vi "playlist.vi"() -> ()   [LabVIEW 2012]
uses:
  System.Windows.Forms
  <vilib>/Utility/miscctls.llb/LVPoint32TypeDef.ctl
  <vilib>/Utility/error.llb/DialogType.ctl
  musicplayer_glo.vi
  <vilib>/Utility/inputDevices.llb/mouseAcquire.vi
  shell32.dll
  user32.dll
panel:
  out "file count":u32
  out "drop-array":string[](array[string])
  out "win msg queue":T1
  in  "cancel":bool
  in  "ProgressBar":refnum<k24>(container)
  out "verdeckung":bool=TRUE
  in  "playlist":i32[](listbox)=[-2] caption="Playlist"
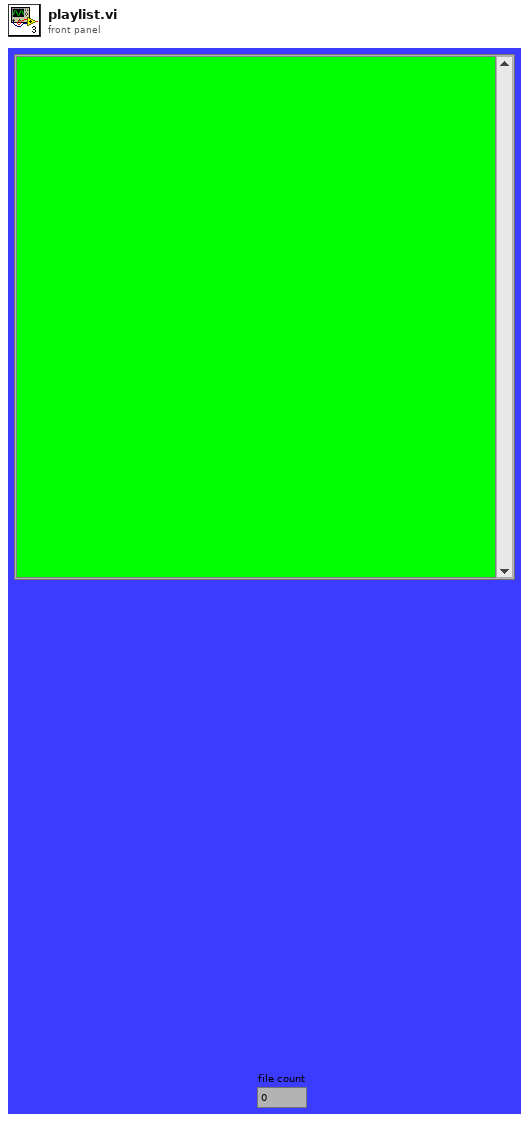
[diagram p1: front panel]
types:
  T1 = typedef "Win Msg Queue RefNum" = refnum<k1>
  T2 = enum8{"Enabled", "Disabled", "Disabled and Grayed Out"}
  T3 = enum32{"Invalid", "Standard", "Closed", "Hidden", "Minimized", "Maximized"}
  T4 = typedef "LVPoint32TypeDef.ctl" = cluster{"Horizontal":i32, "Vertical":i32}
  T5 = cluster{"Horizontal":i32, "Vertical":i32, "Scrolling":i32}
  T6 = cluster{"hWnd":u32, "Msg":u32, "wParam":u32, "lParam":i32, "time":u32, "point":cluster{"X":i32, "Y":i32}}
  T7 = typedef "DialogType.ctl" = u16
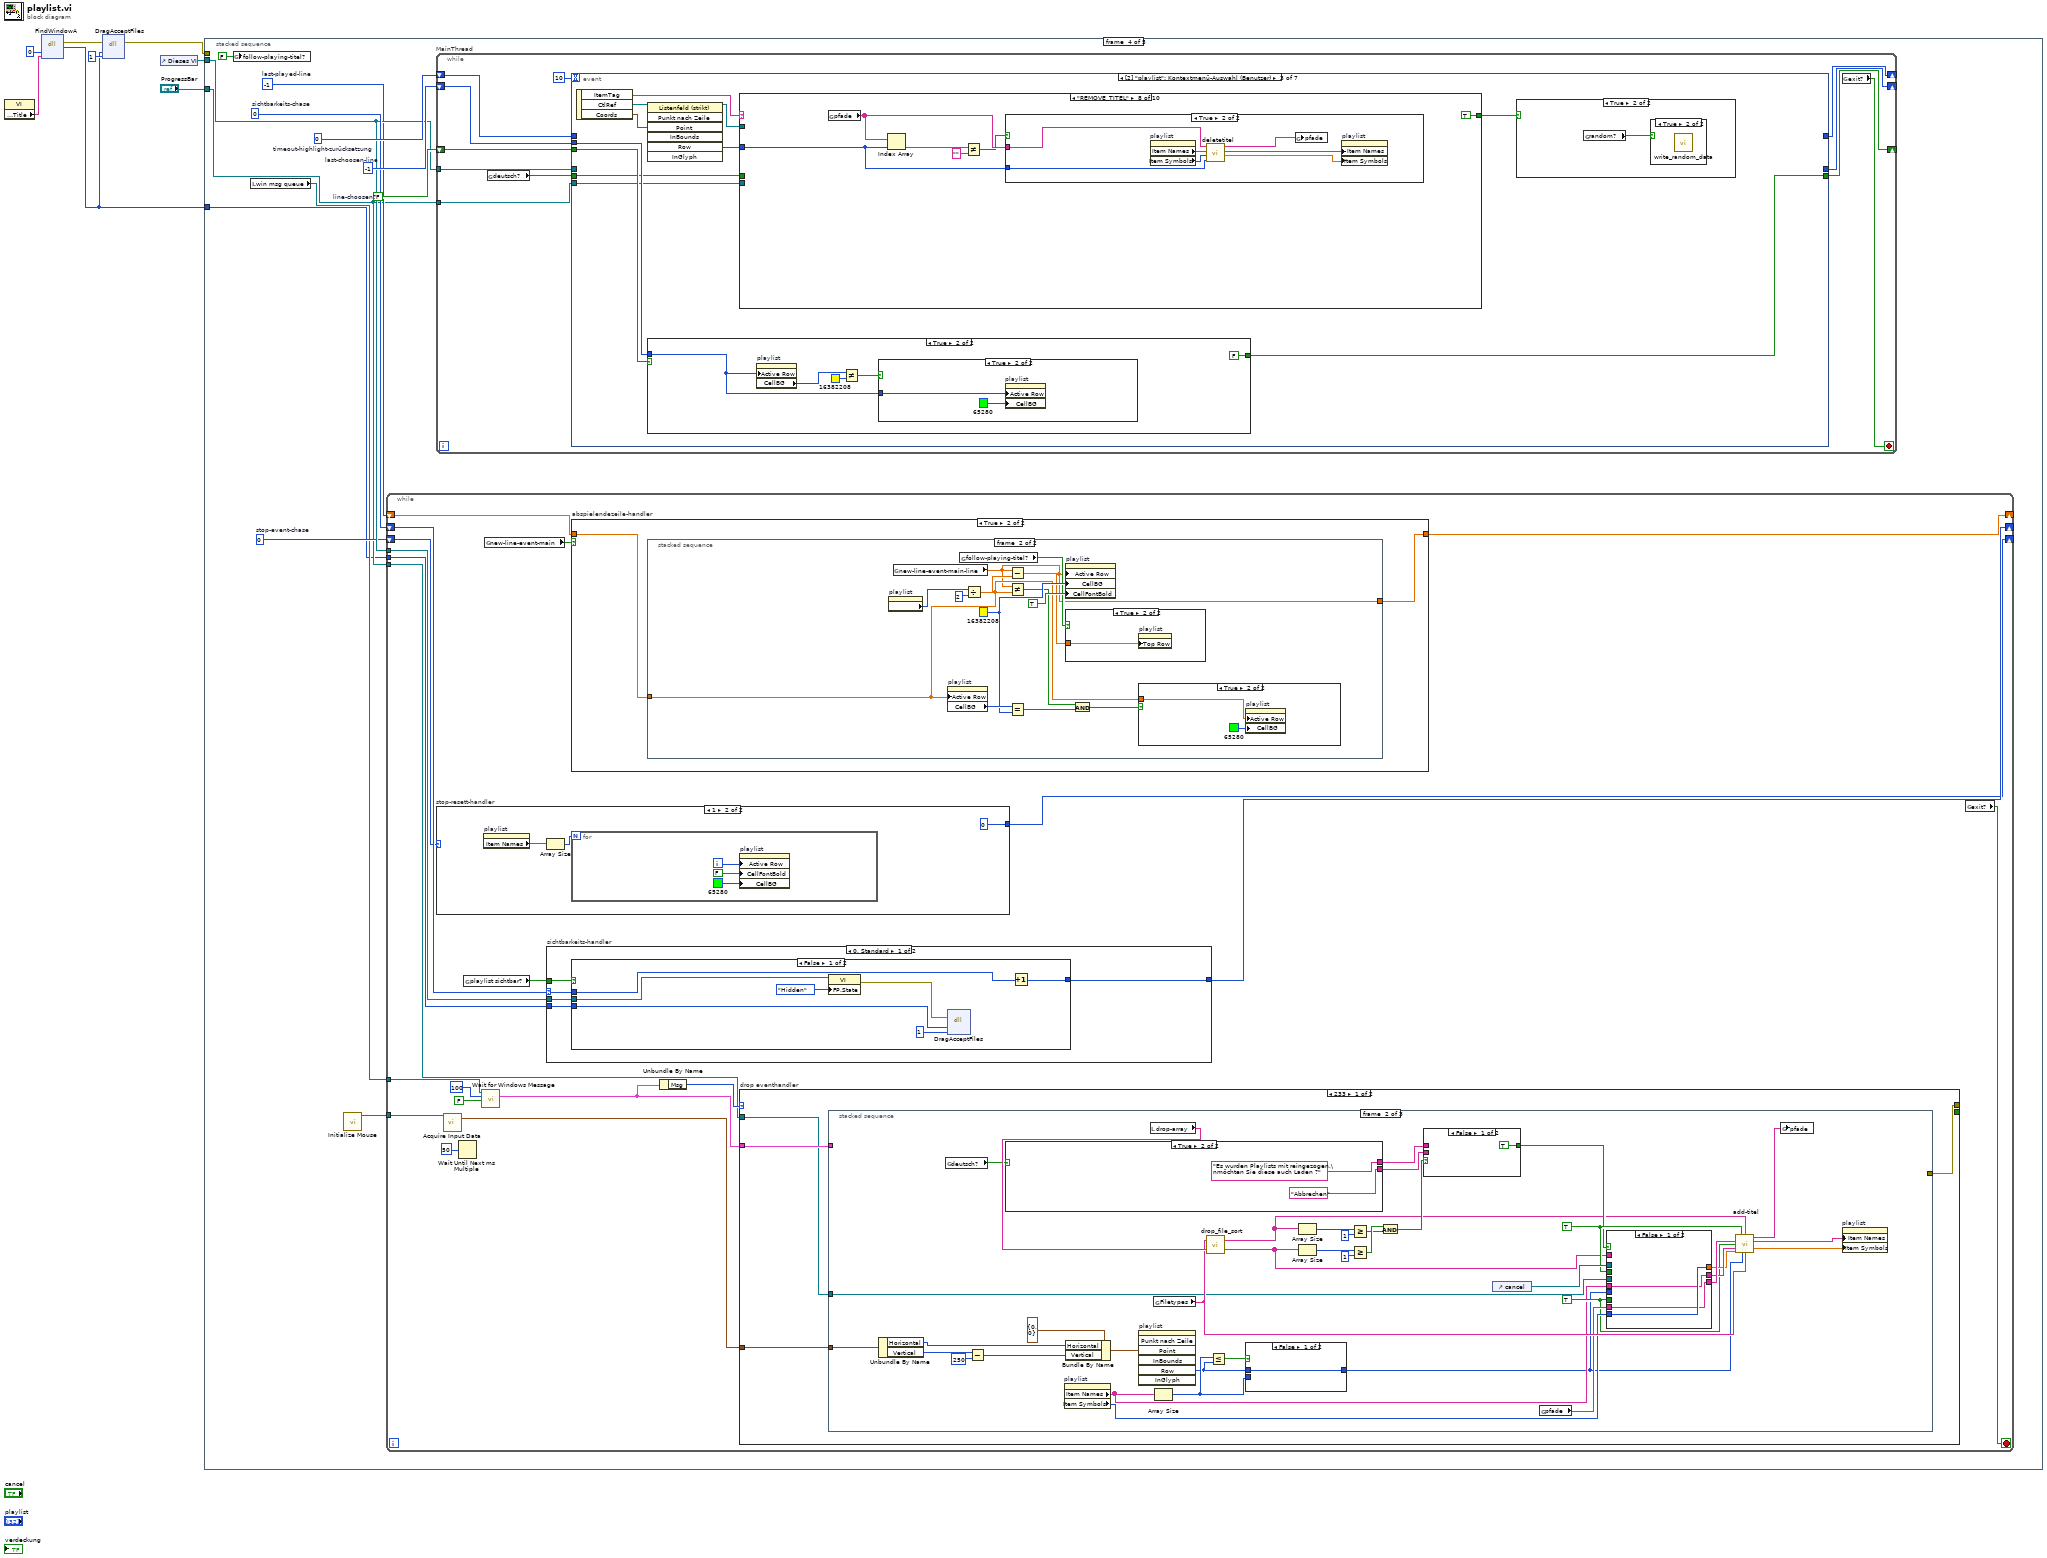
[diagram p0: block diagram]
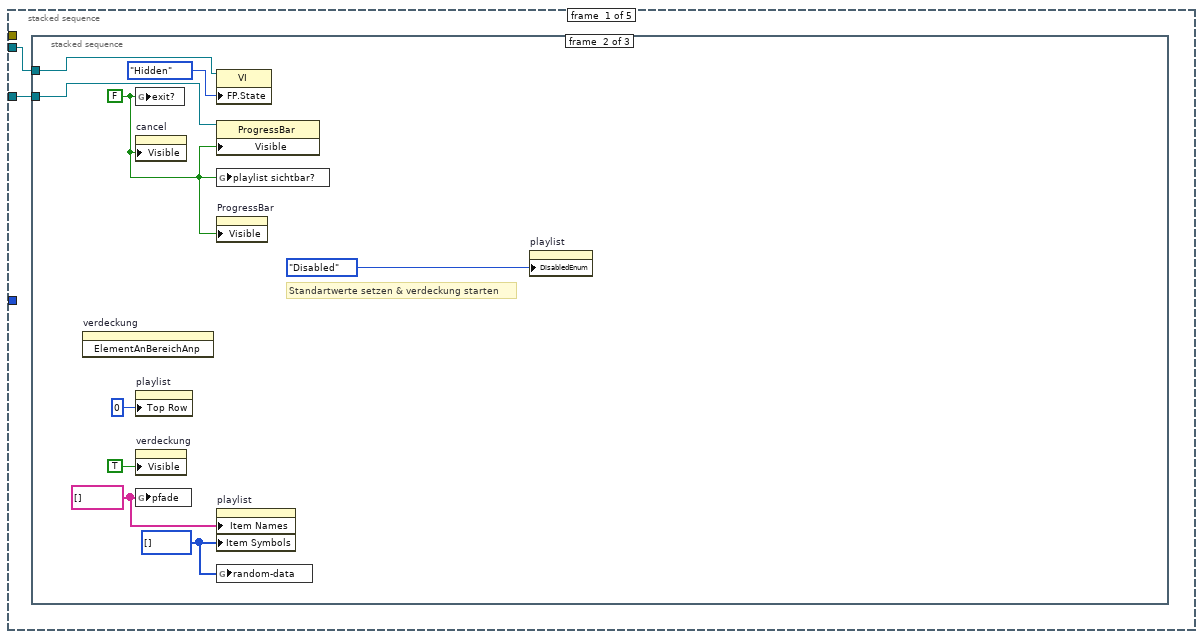
[diagram p2: hidden frame]
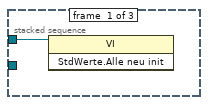
[diagram p3: hidden frame]
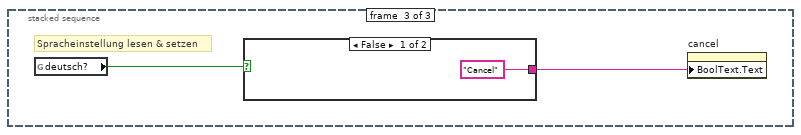
[diagram p4: hidden frame]
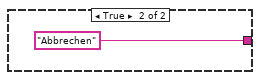
[diagram p5: hidden frame]
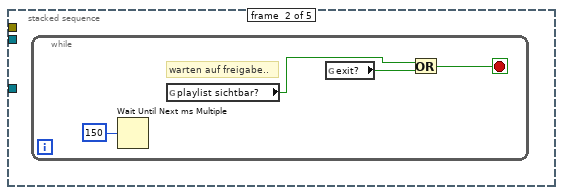
[diagram p6: hidden frame]
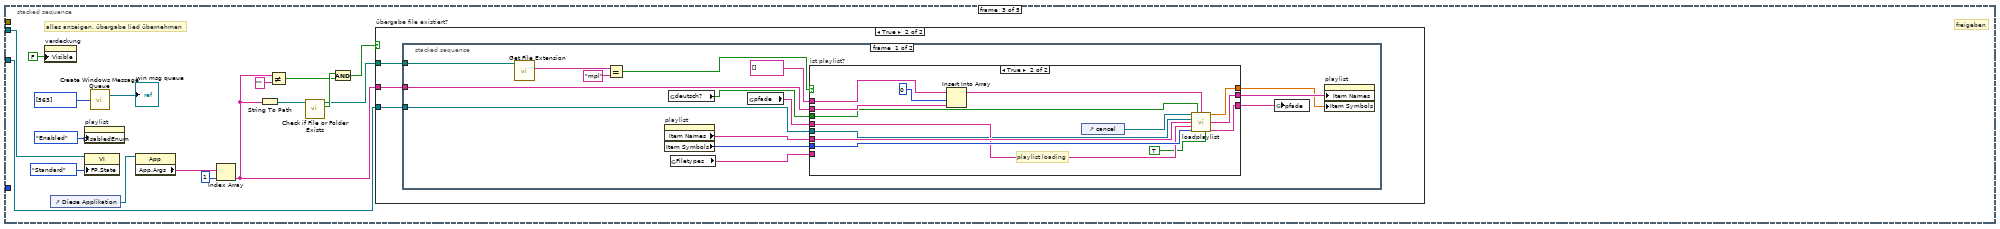
[diagram p7: hidden frame]
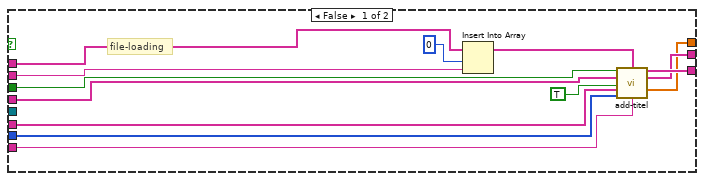
[diagram p9: hidden frame]
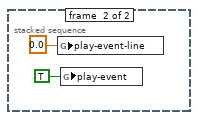
[diagram p10: hidden frame]
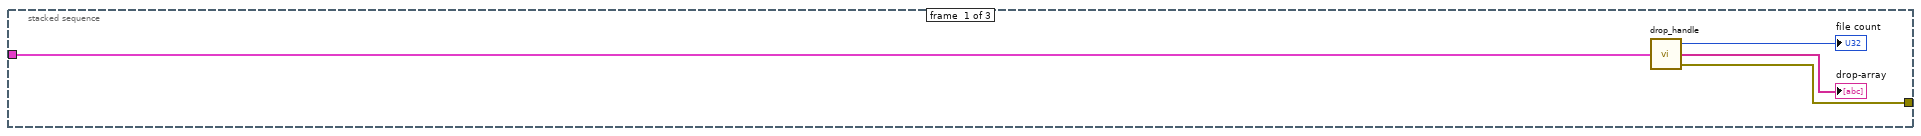
[diagram p11: hidden frame]
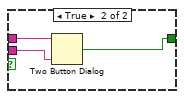
[diagram p12: hidden frame]
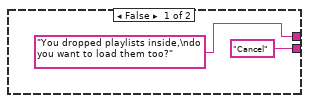
[diagram p13: hidden frame]
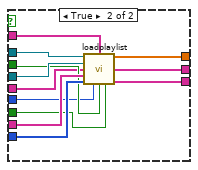
[diagram p14: hidden frame]
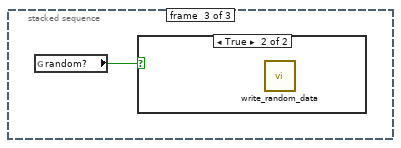
[diagram p16: hidden frame]
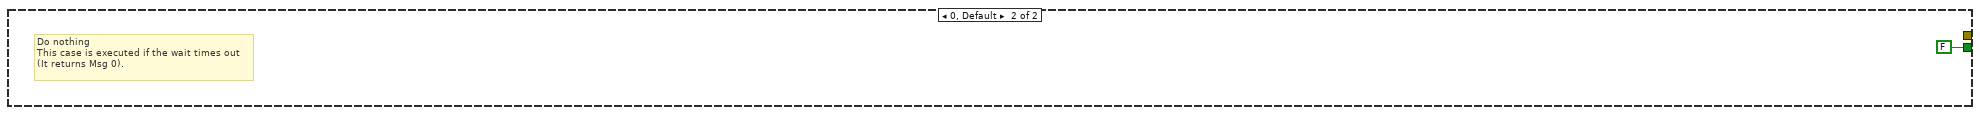
[diagram p18: hidden frame]
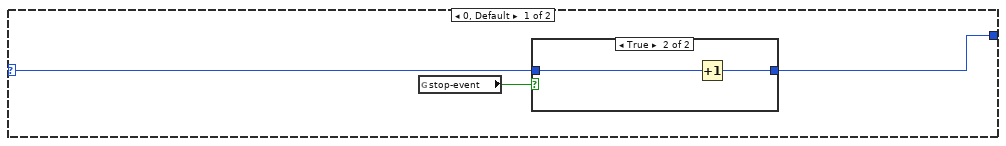
[diagram p19: hidden frame]
diagram:
  n1 = property class="VI"() -> ("Front Panel Window:Title"=w5:string)  [unwired: 2 in, 2 out]
  n2 = dll-call lib="user32.dll" fn="FindWindowA" label="FindWindow"("lpszClassName"=0, "lpszWindowName"=w5) -> (error out=w6:errorcluster, "hWnd"=w1:u32)  [unwired: 5 in, 1 out]
  n3 = dll-call lib="shell32.dll" fn="DragAcceptFiles"(error in=w6, "hWnd"=w1, "fAccept"=1) -> (error out=w2:errorcluster)  [unwired: 5 in, 1 out]
  n4 = control-ref of="Dieses VI"() -> (w8:refnum<vi>)
  n5 = stacked-sequence {
    tunnel: w8 -> [w10 _ w43 w99 w433]
    tunnel: "ProgressBar" -> [w9 _ w29 w94 _]
    tunnel: w2 -> [_ _ _ _ _]
    tunnel: w1 -> [_ _ _ w93 _]
    frame #0 {
      n6 = stacked-sequence {
        tunnel: w10 -> [w11 w17 _]
        tunnel: w9 -> [_ w15 _]
        frame #0 {
          n7 = invoke class="VI" method="StdWerte.Alle neu init"(reference=w11) -> ()  [unwired: 2 in, 3 out]
        }
        frame #1 {
          w12 = i32[] []
          w13 = string[] []
          w14 = FALSE ("playlist sichtbar?")
          # "Standartwerte setzen & verdeckung starten"
          n8 = invoke on="verdeckung" class="Bool." method="ElementAnBereichAnp"() -> ()  [unwired: 3 in, 3 out]
          n9 = global write "musicplayer_glo.vi" "exit?"(w14) -> ()
          n10 = property on="cancel" class="Bool. (strikt)"("Visible"=w14) -> ()  [unwired: 2 in, 2 out]
          n11 = property on="playlist" class="Listenfeld (strikt)"("Top Row"=0 ("Erste Zeile")) -> ()  [unwired: 2 in, 2 out]
          n12 = property on="verdeckung" class="Bool."("Visible"=TRUE ("Sichtbar")) -> ()  [unwired: 2 in, 2 out]
          n13 = global write "musicplayer_glo.vi" "pfade"(w13) -> ()
          n14 = property class="VI"(reference=w17, "FP.State"=T3."Hidden" ("Frontpanel-Fenster:Status")) -> ()  [unwired: 1 in, 2 out]
          n15 = property class="ProgressBar"(reference=w15, "Visible"=w14) -> ()  [unwired: 1 in, 2 out]
          n16 = global write "musicplayer_glo.vi" "playlist sichtbar?"(w14) -> ()
          n17 = property on="ProgressBar" class="AXCont"("Visible"=w14) -> ()  [unwired: 2 in, 2 out]
          n18 = property on="playlist" class="Listenfeld (strikt)"("Item Names"=w13, "Item Symbols"=w12) -> ()  [unwired: 2 in, 2 out]
          n19 = global write "musicplayer_glo.vi" "random-data"(w12) -> ()
          n20 = property on="playlist" class="Listenfeld (strikt)"("DisabledEnum"=T2."Disabled" ("Deaktiviert")) -> ()  [unwired: 2 in, 2 out]
        }
        frame #2 {
          # "Spracheinstellung lesen & setzen"
          n21 = global read "musicplayer_glo.vi" "deutsch?"() -> (w22:bool)
          n22 = case shown="False" w22 {
            tunnel: ["Cancel" "Abbrechen"] -> w21
            frame False {
            }
            frame True {
            }
          }
          n23 = property on="cancel" class="Bool. (strikt)"("BoolText.Text"=w21) -> ()  [unwired: 2 in, 2 out]
        }
      }
    }
    frame #1 {
      n24 = while {
        stop <- w26 stop-if-true
        # "warten auf freigabe.."
        n25 = Wait Until Next ms Multiple(millisecond multiple=u32 150 ("Vielfache von ms")) -> ()  [unwired: 1 out]
        n26 = global read "musicplayer_glo.vi" "playlist sichtbar?"() -> (w27:bool)
        n27 = global read "musicplayer_glo.vi" "exit?"() -> (w25:bool)
        n28 = Or(x=w27, y=w25) -> (x .or. y?=w26:bool)
      }
    }
    frame #2 {
      # "alles anzeigen, übergabe lied übernehmen"
      # "freigeben"
      n29 = property on="verdeckung" class="Bool."("Visible"=FALSE ("Sichtbar")) -> ()  [unwired: 2 in, 2 out]
      n30 = control-ref of="Diese Applikation"() -> (w39:refnum<vi>)
      n31 = property on="playlist" class="Listenfeld (strikt)"("DisabledEnum"=T2."Enabled" ("Deaktiviert")) -> ()  [unwired: 2 in, 2 out]
      n32 = property class="VI"(reference=w43, "FP.State"=T3."Standard" ("Frontpanel-Fenster:Status")) -> ()  [unwired: 1 in, 2 out]
      n33 = call "Create Windows Message Queue.vi"("Messeges (none)"=u32[] [563]) -> ("win msg queue"=→"win msg queue":T1)  [unwired: 2 in, 1 out]
      n34 = property class="App"(reference=w39) -> ("App.Args"=w38:string[])  [unwired: 1 in, 2 out]
      n35 = Index Array(array=w38, index=1 ("Index")) -> (element=w33:string)
      n36 = String To Path(string=w33) -> (path=w36:path)
      n37 = Not Equal?(x=w33, y="") -> (x != y?=w30:bool)
      n38 = call <vilib>:"Check if File or Folder Exists.vi"("path"=w36) -> ("file or folder exists?"=w35:bool, "dup path"=w34:path)  [unwired: 8 in, 1 out]
      n39 = And(x=w35, y=w30) -> (x .and. y?=w31:bool)
      n40 = case "übergabe file existiert?" shown="True" w31 {
        tunnel: w34 -> [_ w48]
        tunnel: w33 -> [_ w47]
        tunnel: w29 -> [_ w46]
        frame False {
        }
        frame True {
          n41 = stacked-sequence {
            tunnel: w48 -> [w63 _]
            tunnel: w47 -> [w55 _]
            tunnel: w46 -> [w49 _]
            frame #0 {
              n42 = call <vilib>:"Get File Extension.vi"("file"=w63) -> ("lowercase file extension"=w62:string)  [unwired: 7 in, 3 out]
              n43 = Equal?(x=w62, y="mpl") -> (x = y?=w60:bool)
              n44 = property on="playlist" class="Listenfeld (strikt)"() -> ("Item Names"=w57:string[], "Item Symbols"=w56:i32[])  [unwired: 2 in, 2 out]
              n45 = global read "musicplayer_glo.vi" "deutsch?"() -> (w59:bool)
              n46 = global read "musicplayer_glo.vi" "Filetypes"() -> (w54:string)
              n47 = global read "musicplayer_glo.vi" "pfade"() -> (w58:string[])
              n48 = case "ist playlist?" shown="True" w60 {
                tunnel: w59 -> [w76 w86]
                tunnel: w58 -> [w75 w83]
                tunnel: w57 -> [w73 w85]
                tunnel: w56 -> [w72 w84]
                tunnel: w55 -> [w70 w88]
                tunnel: w54 -> [w68 _]
                tunnel: [w67 w81] -> w53
                tunnel: [w66 w80] -> w52
                tunnel: [w65 w79] -> w51
                tunnel: string[] [] -> [w64 w89]
                tunnel: w49 -> [_ w78]
                frame False {
                  # "file-loading"
                  n49 = Insert Into Array(array=w64, index=0 ("Index"), new element=w70) -> (w69:string[])
                  n50 = call "add-titel.vi"("deutsch?"=w76, "input-array"=w69, "pfade"=w75, "use input-array?"=TRUE, "playlist"=w73, "symbole"=w72, "dateitypen"=w68) -> ("pfade out"=w67:string[], "playlist out"=w66:string[], "symbole out"=w65:dbl[])  [unwired: 6 in]
                }
                frame True {
                  # "playlist loading"
                  n51 = Insert Into Array(array=w89, index=0 ("Index"), new element=w88) -> (w87:string[])
                  n52 = control-ref of="cancel"() -> (w77:refnum<vi>)
                  n53 = call "loadplaylist.vi"("Boolesch-ref"=w77, "deutsch?"=w86, "input-array"=w87, "ProgressBar-ref"=w78, "playlist-input"=w85, "pfade-in"=w83, "symbole-in"=w84, "von input-array?"=TRUE) -> ("symbole-out"=w79:dbl[], "playlist-output"=w80:string[], "pfade-out"=w81:string[])  [unwired: 5 in]
                }
              }
              n54 = global write "musicplayer_glo.vi" "pfade"(w53) -> ()
              n55 = property on="playlist" class="Listenfeld (strikt)"("Item Names"=w52, "Item Symbols"=w51) -> ()  [unwired: 2 in, 2 out]
            }
            frame #1 {
              n56 = global write "musicplayer_glo.vi" "play-event-line"(0.0 ("play-event-line")) -> ()
              n57 = global write "musicplayer_glo.vi" "play-event"(TRUE ("play-event-playlist")) -> ()
            }
          }
        }
      }
    }
    frame #3 {
      w97 = 0  # stop-event-chase
      w98 = -1  # last-played-line
      w100 = 0  # sichtbarkeits-chase
      w102 = 0  # timeout-highlight-zurücksetzung
      w103 = FALSE  # line-choosen?
      w104 = -1  # last-choosen-line
      n58 = global write "musicplayer_glo.vi" "follow-playing-titel?"(FALSE ("follow-playing-titel?")) -> ()
      n59 = local read "win msg queue"() -> (w96:T1)
      n60 = call <vilib>:"Initialize Mouse.vi"() -> ("device ID"=w95:refnum<k1>)  [unwired: 10 in, 1 out]
      n61 = while {
        shift-right: [w120] -> _
        shift-left: w100 -> [w122]
        tunnel: w99 -> [w121]
        shift-right: [w117] -> _
        shift-left: w98 -> [w118]
        shift-right: [w115] -> _
        shift-left: w97 -> [w116]
        tunnel: w96 -> [w109]
        tunnel: w95 -> [w108]
        tunnel: w94 -> [w107]
        tunnel: w93 -> [w105]
        stop <- w106 stop-if-true
        n62 = case "stop-resett-handler" shown="1" w116 {
          selector: w116 -> [w200 _]
          tunnel: [w199 0] -> w115
          frame 0, Default {
            n63 = global read "musicplayer_glo.vi" "stop-event"() -> (w201:bool)
            n64 = case shown="True" w201 {
              tunnel: w200 -> [w202 w204]
              tunnel: [w202 w203] -> w199
              frame False {
              }
              frame True {
                n65 = Increment(x=w204) -> (x+1=w203:i32)
              }
            }
          }
          frame 1 {
            n66 = property on="playlist" class="Listenfeld (strikt)"() -> ("Item Names"=w207:string[])  [unwired: 2 in, 2 out]
            n67 = Array Size(array=w207) -> (size(s)=w206:i32)
            n68 = for {
              N: w206 -> [_]
              i -> [w209]
              n69 = property on="playlist" class="Listenfeld (strikt)"("Active Row"=w209, "CellFontBold"=FALSE ("Aktive Zeile:Schriftart der Zelle:Fett"), "CellBG"=u32 65280 ("Farbfeld 2")) -> ()  [unwired: 2 in, 2 out]
            }
          }
        }
        n70 = call-poly <vilib>:"Acquire Input Data.vi"("device ID"=w108) -> ("axis info"=w112:T5)  [unwired: 15 in, 3 out]
        n71 = Wait Until Next ms Multiple(millisecond multiple=u32 50 ("Vielfache von ms")) -> ()  [unwired: 1 out]
        n72 = global read "musicplayer_glo.vi" "playlist sichtbar?"() -> (w123:bool)
        n73 = call "Wait for Windows Message.vi"("win msg queue"=w109, "ms timeout (-1)"=100, "ignore previous (F)"=FALSE ("ignore previous (T)")) -> ("Message"=w111:T6)  [unwired: 1 in, 5 out]
        n74 = global read "musicplayer_glo.vi" "new-line-event-main"() -> (w119:bool)
        n75 = case "sichtbarkeits-handler" shown="0, Standard" w122 {
          selector: w122 -> [w234 w246]
          tunnel: w123 -> [w235 w248]
          tunnel: [w233 w247] -> w120
          tunnel: w121 -> [w232 w245]
          tunnel: w105 -> [w231 w244]
          frame 0, Default {
            n76 = case shown="False" w235 {
              tunnel: w234 -> [w240 w243]
              tunnel: [w239 w243] -> w233
              tunnel: w232 -> [w242 _]
              tunnel: w231 -> [w237 _]
              frame False {
                n77 = property class="VI"(reference=w242, "FP.State"=T3."Hidden" ("Frontpanel-Fenster:Status")) -> (error out=w236:errorcluster)  [unwired: 1 in, 1 out]
                n78 = dll-call lib="shell32.dll" fn="DragAcceptFiles"(error in=w236, "hWnd"=w237, "fAccept"=1) -> ()  [unwired: 5 in, 2 out]
                n79 = Increment(x=w240) -> (x+1=w239:i32)
              }
              frame True {
              }
            }
          }
          frame 1 {
            n80 = case shown="True" w248 {
              tunnel: [w249 0] -> w247
              tunnel: w246 -> [w249 _]
              tunnel: w245 -> [_ w253]
              tunnel: w244 -> [_ w251]
              frame False {
              }
              frame True {
                n81 = property class="VI"(reference=w253, "FP.State"=T3."Standard" ("Frontpanel-Fenster:Status")) -> (error out=w250:errorcluster)  [unwired: 1 in, 1 out]
                n82 = dll-call lib="shell32.dll" fn="DragAcceptFiles"(error in=w250, "hWnd"=w251, "fAccept"=1) -> ()  [unwired: 5 in, 2 out]
              }
            }
          }
        }
        n83 = case "abspielendezeile-handler" shown="True" w119 {
          tunnel: w118 -> [w211 w213]
          tunnel: [w211 w212] -> w117
          frame False {
          }
          frame True {
            n84 = stacked-sequence {
              tunnel: w213 -> [_ w216]
              tunnel: [_ w215] -> w212
              frame #0 {
                n85 = global write "musicplayer_glo.vi" "new-line-event-main"(FALSE ("new-line-event-main")) -> ()
              }
              frame #1 {
                w223 = u32 16382208 ("Farbfeld 2")
                n86 = property on="playlist" class="Listenfeld (strikt)"() -> ("Number of Rows"=w221:u32)  [unwired: 2 in, 2 out]
                n87 = global read "musicplayer_glo.vi" "new-line-event-main-line"() -> (w215:dbl)
                n88 = property on="playlist" class="Listenfeld (strikt)"("Active Row"=w216) -> ("CellBG"=w227:u32)  [unwired: 2 in, 2 out]
                n89 = global read "musicplayer_glo.vi" "follow-playing-titel?"() -> (w218:bool)
                n90 = Divide(x=w221, y=u32 2) -> (x/y=w217:dbl)
                n91 = Subtract(x=w215, y=w217) -> (x-y=w219:dbl)
                n92 = Not Equal?(x=w215, y=w216) -> (x != y?=w222:bool)
                n93 = Equal?(x=w227, y=w223) -> (x = y?=w226:bool)
                n94 = property on="playlist" class="Listenfeld (strikt)"("Active Row"=w215, "CellBG"=w223, "CellFontBold"=TRUE ("Aktive Zeile:Schriftart der Zelle:Fett")) -> ()  [unwired: 2 in, 2 out]
                n95 = case shown="True" w218 {
                  tunnel: w219 -> [_ w228]
                  frame False {
                  }
                  frame True {
                    n96 = property on="playlist" class="Listenfeld (strikt)"("Top Row"=w228) -> ()  [unwired: 2 in, 2 out]
                  }
                }
                n97 = And(x=w222, y=w226) -> (x .and. y?=w224:bool)
                n98 = case shown="True" w224 {
                  tunnel: w216 -> [_ w230]
                  frame False {
                  }
                  frame True {
                    n99 = property on="playlist" class="Listenfeld (strikt)"("Active Row"=w230, "CellBG"=u32 65280 ("Farbfeld 2")) -> ()  [unwired: 2 in, 2 out]
                  }
                }
              }
            }
          }
        }
        n100 = Unbundle By Name(w111) -> ("Msg"=w110:u32)
        n101 = case "drop eventhandler" shown="233" w110 {
          tunnel: [_ FALSE] -> _
          tunnel: [w127 _] -> _
          tunnel: w111 -> [w128 _]
          tunnel: w107 -> [w126 _]
          tunnel: w112 -> [w125 _]
          frame 563 {
            n102 = stacked-sequence {
              tunnel: [w132 _ _] -> w127
              tunnel: w128 -> [w131 _ _]
              tunnel: w126 -> [_ w165 _]
              tunnel: w125 -> [_ w146 _]
              frame #0 {
                n103 = call "drop_handle.vi"("Message"=w131) -> ("error out"=w132:errorcluster, "drop-array"=→"drop-array":string[], "file count"=→"file count":u32)
              }
              frame #1 {
                w158 = TRUE ("ab position?")
                w159 = TRUE ("use input-array?")
                n104 = Unbundle By Name(w146) -> ("Horizontal"=w152:i32, "Vertical"=w150:i32)
                n105 = global read "musicplayer_glo.vi" "deutsch?"() -> (w142:bool)
                n106 = Subtract(x=w150, y=250) -> (x-y=w149:i32)
                n107 = case shown="True" w142 {
                  tunnel: ["You dropped playlists inside,\ndo you want to load them too?" "Es wurden Playlists mit reingezogen,\nmöchten Sie diese auch Laden ?"] -> w140
                  tunnel: ["Cancel" "Abbrechen"] -> w141
                  frame False {
                  }
                  frame True {
                  }
                }
                n108 = property on="playlist" class="Listenfeld (strikt)"() -> ("Item Names"=w157:string[], "Item Symbols"=w160:i32[])  [unwired: 2 in, 2 out]
                n109 = Bundle By Name(cluster=T4 {"Horizontal"=0, "Vertical"=0} ("Koordinaten"), "Horizontal"=w152, "Vertical"=w149) -> (w147:T4)
                n110 = invoke on="playlist" class="Listenfeld (strikt)" method="Punkt nach Zeile"("Point"=w147) -> ("Row"=w153:i32)  [unwired: 6 in, 6 out]
                n111 = local read "drop-array"() -> (w171:string[])
                n112 = global read "musicplayer_glo.vi" "Filetypes"() -> (w167:string)
                n113 = Array Size(array=w157) -> (size(s)=w156:i32)
                n114 = call "drop_file_sort.vi"("drop-array"=w171, "filetypes"=w167) -> ("playlist-array"=w145:string[], "file-array"=w133:string[])
                n115 = Less Or Equal?(x=w156, y=w153) -> (x <= y?=w155:bool)
                n116 = case shown="False" w155 {
                  tunnel: w156 -> [_ w196]
                  tunnel: [w195 w196] -> w154
                  tunnel: w153 -> [w195 _]
                  frame False {
                  }
                  frame True {
                  }
                }
                n117 = Array Size(array=w133) -> (size(s)=w137:i32)
                n118 = Array Size(array=w145) -> (size(s)=w144:i32)
                n119 = Greater Or Equal?(x=w137, y=1) -> (x >= y?=w134:bool)
                n120 = Greater Or Equal?(x=w144, y=1) -> (x >= y?=w139:bool)
                n121 = And(x=w139, y=w134) -> (x .and. y?=w135:bool)
                n122 = case shown="False" w135 {
                  tunnel: w141 -> [_ w175]
                  tunnel: w140 -> [_ w174]
                  tunnel: [TRUE ("T button?") w173] -> w138
                  frame False {
                  }
                  frame True {
                    n123 = Two Button Dialog(message=w174, 1:w175) -> (T button?=w173:bool)  [unwired: 1 in]
                  }
                }
                n124 = control-ref of="cancel"() -> (w166:refnum<vi>)
                n125 = global read "musicplayer_glo.vi" "pfade"() -> (w164:string[])
                n126 = case shown="False" w138 {
                  tunnel: w166 -> [_ w194]
                  tunnel: w165 -> [_ w193]
                  tunnel: w164 -> [w180 w192]
                  tunnel: [w180 w191] -> w163
                  tunnel: [w181 w190] -> w162
                  tunnel: [w182 w189] -> w161
                  tunnel: w160 -> [w182 w188]
                  tunnel: w145 -> [_ w187]
                  tunnel: w159 -> [_ w186]
                  tunnel: w158 -> [_ w185]
                  tunnel: w157 -> [w181 w184]
                  tunnel: w154 -> [_ w183]
                  frame False {
                  }
                  frame True {
                    n127 = call "loadplaylist.vi"("Boolesch-ref"=w194, "input-array"=w187, "ProgressBar-ref"=w193, "playlist-input"=w184, "pfade-in"=w192, "symbole-in"=w188, "ab position"=w183, "ab position?"=w185, "von input-array?"=w186) -> ("symbole-out"=w189:dbl[], "playlist-output"=w190:string[], "pfade-out"=w191:string[])  [unwired: 4 in]
                  }
                }
                n128 = call "add-titel.vi"("abposeinfügen"=w158, "input-array"=w133, "pfade"=w163, "use input-array?"=w159, "playlist"=w162, "symbole"=w161, "pos"=w154, "dateitypen"=w167) -> ("pfade out"=w170:string[], "playlist out"=w169:string[], "symbole out"=w168:dbl[])  [unwired: 5 in]
                n129 = global write "musicplayer_glo.vi" "pfade"(w170) -> ()
                n130 = property on="playlist" class="Listenfeld (strikt)"("Item Names"=w169, "Item Symbols"=w168) -> ()  [unwired: 2 in, 2 out]
              }
              frame #2 {
                n131 = global read "musicplayer_glo.vi" "random?"() -> (w197:bool)
                n132 = case shown="True" w197 {
                  frame False {
                  }
                  frame True {
                    n133 = call "write_random_data.vi"() -> ()  [unwired: 12 in]
                  }
                }
              }
            }
          }
          frame 0, Default {
            # "Do nothing\nThis case is executed if the wait times out\n(It returns Msg 0)."
          }
        }
        n134 = global read "musicplayer_glo.vi" "exit?"() -> (w106:bool)
      }
      n135 = while "MainThread" {
        tunnel: w99 -> [w258]
        shift-right: [w263] -> _
        shift-left: w103 -> [w265]
        shift-right: [w264] -> _
        shift-left: w104 -> [w266]
        tunnel: w94 -> [w257]
        shift-right: [w259] -> _
        shift-left: w102 -> [w260]
        stop <- w261 stop-if-true
        n136 = global read "musicplayer_glo.vi" "deutsch?"() -> (w262:bool)
        n137 = event "Ereignisstruktur" shown="[2] \"playlist\": Kontextmenü-Auswahl (Benutzer)" {
          selector: _ -> [_ _ _ _ _ _ _]
          dyn-events: _ -> [_ _ _ _ _ _ _]
          timeout: 10 -> [_ _ _ _ _ _ _]
          tunnel: w258 -> [_ _ _ _ _ _ _]
          tunnel: w266 -> [_ _ w315 _ w411 w423 w430]
          tunnel: w265 -> [_ _ w314 _ w412 w422 w429]
          tunnel: [_ w283 _ _ _ w423 w430] -> w264
          tunnel: [_ TRUE w313 _ w410 w422 w429] -> w263
          tunnel: w257 -> [_ _ w311 _ _ _ _]
          tunnel: w262 -> [_ _ w306 _ _ _ _]
          tunnel: w260 -> [_ _ _ _ _ w421 _]
          tunnel: [_ _ _ _ _ w420 _] -> w259
          event "playlist": Double Click {
            n138 = event-data() -> ("Coords"=w269:T4, "CtlRef"=w270:refnum<vi>)  [unwired: 1 in]
            n139 = invoke class="Listenfeld (strikt)" method="Punkt nach Zeile"(reference=w270, "Point"=w269) -> ("Row"=w268:i32)  [unwired: 5 in, 6 out]
            n140 = global read "musicplayer_glo.vi" "pfade"() -> (w273:string[])
            n141 = Index Array(array=w273, index=w268) -> (element=w271:string)
            n142 = Not Equal?(x=w271, y="") -> (x != y?=w267:bool)
            n143 = case shown="True" w267 {
              tunnel: w270 -> [_ w275]
              tunnel: w268 -> [_ w274]
              frame False {
              }
              frame True {
                n144 = stacked-sequence {
                  tunnel: w275 -> [_ _]
                  tunnel: w274 -> [w277 _]
                  frame #0 {
                    n145 = global write "musicplayer_glo.vi" "play-event-line"(w277) -> ()
                    n146 = property on="playlist" class="Listenfeld (strikt)"() -> ("Item Symbols"=w279:i32[])  [unwired: 2 in, 2 out]
                    n147 = Replace Array Subset(array=w279, new element=38, index=w277) -> (w278:i32[])
                    n148 = property on="playlist" class="Listenfeld (strikt)"("Item Symbols"=w278) -> ()  [unwired: 2 in, 2 out]
                  }
                  frame #1 {
                    n149 = global write "musicplayer_glo.vi" "play-event"(TRUE ("play-event-playlist")) -> ()
                  }
                }
              }
            }
          }
          event "playlist": Shortcut Menu Activation? {
            w292 = T7 0 items=["no dialog", "OK message", "continue or stop message", "OK message + warnings", "continue/stop + warnings"] ("type of dialog (OK msg:1)")
            n150 = event-data() -> ("MenuRef"=w301:refnum<k9>, "Coords"=w299:T4, "CtlRef"=w297:refnum<vi>)  [unwired: 1 in]
            n151 = invoke class="Listenfeld (strikt)" method="Punkt nach Zeile"(reference=w297, "Point"=w299) -> (reference out=w286:refnum<vi>, "Row"=w283:i32)  [unwired: 5 in, 5 out]
            n152 = property class="Listenfeld (strikt)"(reference=w297) -> ("Item Names"=w298:string[])  [unwired: 1 in, 2 out]
            n153 = property class="Listenfeld (strikt)"(reference=w286, "Active Row"=w283) -> (reference out=w285:refnum<vi>, "CellBG"=w284:u32)  [unwired: 1 in, 1 out]
            n154 = Index Array(array=w298, index=w283) -> (element=w296:string)
            n155 = Not Equal?(x=w296, y="") -> (x != y?=w294:bool)
            n156 = Not Equal?(x=w284, y=u32 16382208 ("Farbfeld 2")) -> (x != y?=w282:bool)
            n157 = global read "musicplayer_glo.vi" "follow-playing-titel?"() -> (w287:bool)
            n158 = case shown="False" w282 {
              tunnel: w285 -> [_ w303]
              tunnel: w283 -> [_ w302]
              frame False {
              }
              frame True {
                n159 = property class="Listenfeld (strikt)"(reference=w303, "Active Row"=w302, "CellBG"=u32 13816530 ("Farbfeld 2")) -> ()  [unwired: 1 in, 2 out]
              }
            }
            n160 = Set Menu Item Info(7:"REMOVE_TITEL" ("Menüpunkt-Tag"), 9:w294, 11:w301) -> (0:w289:errorcluster, 3:w290:refnum<k9>)  [unwired: 2 in, 2 out]
            n161 = Set Menu Item Info(6:w287, 7:"FOLLOW_PLAY", 8:w289, 11:w290) -> (0:w288:errorcluster)  [unwired: 2 in, 2 out]
            n162 = call <vilib>:"Simple Error Handler.vi"("type of dialog (OK msg:1)"=w292, "error in (no error)"=w288) -> ()  [unwired: 1 in, 7 out]
            n163 = event-data() -> ()  [unwired: 2 in, 1 out]
          }
          event "playlist": Shortcut Menu Selection (User) {
            n164 = event-data() -> ("ItemTag"=w312:string, "CtlRef"=w308:refnum<vi>, "Coords"=w310:T4)  [unwired: 1 in]
            n165 = invoke class="Listenfeld (strikt)" method="Punkt nach Zeile"(reference=w308, "Point"=w310) -> (reference out=w307:refnum<vi>, "Row"=w309:i32)  [unwired: 5 in, 5 out]
            n166 = case shown="True" w314 {
              tunnel: w315 -> [_ w394]
              tunnel: [_ FALSE] -> w313
              frame False {
              }
              frame True {
                n167 = property on="playlist" class="Listenfeld (strikt)"("Active Row"=w394) -> ("CellBG"=w396:u32)  [unwired: 2 in, 2 out]
                n168 = Not Equal?(x=w396, y=u32 16382208 ("Farbfeld 2")) -> (x != y?=w395:bool)
                n169 = case shown="True" w395 {
                  tunnel: w394 -> [_ w398]
                  frame False {
                  }
                  frame True {
                    n170 = property on="playlist" class="Listenfeld (strikt)"("Active Row"=w398, "CellBG"=u32 65280 ("Farbfeld 2")) -> ()  [unwired: 2 in, 2 out]
                  }
                }
              }
            }
            n171 = case shown="\"REMOVE_TITEL\"" w312 {
              tunnel: [FALSE TRUE _ _ TRUE TRUE _ TRUE TRUE _] -> w305
              tunnel: w311 -> [_ w321 _ _ _ _ _ _ _ _]
              tunnel: w309 -> [_ w320 _ w346 _ w360 _ w372 _ _]
              tunnel: w307 -> [_ _ _ _ _ _ _ _ _ _]
              tunnel: w306 -> [_ w319 w341 _ _ w368 _ _ _ _]
              frame "default", Default {
              }
              frame "LOAD_PLAYLIST" {
                n172 = stacked-sequence {
                  tunnel: w321 -> [w324 w331 w340]
                  tunnel: w320 -> [_ w327 _]
                  tunnel: w319 -> [_ _ _]
                  frame #0 {
                    w322 = TRUE ("Sichtbar")
                    # "show cancel & statbar"
                    n173 = property on="ProgressBar" class="AXCont"("Visible"=w322) -> ()  [unwired: 2 in, 2 out]
                    n174 = property on="cancel" class="Bool. (strikt)"("Visible"=w322) -> ()  [unwired: 2 in, 2 out]
                    n175 = property on="verdeckung" class="Bool."("Visible"=w322) -> ()  [unwired: 2 in, 2 out]
                    n176 = property class="ProgressBar"(reference=w324, "Visible"=w322, "Value"=0) -> ()  [unwired: 1 in, 2 out]
                  }
                  frame #1 {
                    # "load playlist via subvi"
                    n177 = global read "musicplayer_glo.vi" "pfade"() -> (w338:string[])
                    n178 = Index Array(array=w338, index=w327) -> (element=w337:string)
                    n179 = global read "musicplayer_glo.vi" "deutsch?"() -> (w330:bool)
                    n180 = property on="playlist" class="Listenfeld (strikt)"() -> ("Item Names"=w332:string[], "Item Symbols"=w333:i32[])  [unwired: 2 in, 2 out]
                    n181 = control-ref of="cancel"() -> (w335:refnum<vi>)
                    n182 = Not Equal?(x=w337, y="") -> (x != y?=w328:bool)
                    n183 = global read "musicplayer_glo.vi" "pfade"() -> (w334:string[])
                    n184 = call "loadplaylist.vi"("Boolesch-ref"=w335, "deutsch?"=w330, "ProgressBar-ref"=w331, "playlist-input"=w332, "pfade-in"=w334, "symbole-in"=w333, "ab position"=w327, "ab position?"=w328) -> ("symbole-out"=w329:dbl[], "playlist-output"=w325:string[], "pfade-out"=w326:string[])  [unwired: 5 in]
                    n185 = global write "musicplayer_glo.vi" "pfade"(w326) -> ()
                    n186 = property on="playlist" class="Listenfeld (strikt)"("Item Names"=w325, "Item Symbols"=w329) -> ()  [unwired: 2 in, 2 out]
                  }
                  frame #2 {
                    w339 = FALSE
                    n187 = property on="cancel" class="Bool. (strikt)"("Visible"=w339) -> ()  [unwired: 2 in, 2 out]
                    n188 = property class="ProgressBar"(reference=w340, "Visible"=w339) -> ()  [unwired: 1 in, 2 out]
                    n189 = property on="ProgressBar" class="AXCont"("Visible"=w339) -> ()  [unwired: 2 in, 2 out]
                    n190 = property on="verdeckung" class="Bool."("Visible"=w339) -> ()  [unwired: 2 in, 2 out]
                  }
                }
              }
              frame "SAVE_PLAYLIST" {
                n191 = global read "musicplayer_glo.vi" "pfade"() -> (w342:string[])
                n192 = call "saveplaylist.vi"("pfade"=w342, "deutsch?"=w341) -> ()  [unwired: 10 in]
              }
              frame "PLAY_TITEL" {
                n193 = global read "musicplayer_glo.vi" "pfade"() -> (w347:string[])
                n194 = Index Array(array=w347, index=w346) -> (element=w345:string)
                n195 = Not Equal?(x="" ("Element"), y=w345) -> (x != y?=w343:bool)
                n196 = case shown="True" w343 {
                  tunnel: w346 -> [_ w348]
                  frame False {
                  }
                  frame True {
                    n197 = stacked-sequence {
                      tunnel: w348 -> [w349 _]
                      frame #0 {
                        n198 = global write "musicplayer_glo.vi" "play-event-line"(w349) -> ()
                      }
                      frame #1 {
                        n199 = global write "musicplayer_glo.vi" "play-event"(TRUE ("play-event-playlist")) -> ()
                      }
                    }
                  }
                }
              }
              frame "CLEAR_PLAYLIST" {
                n200 = stacked-sequence {
                  frame #0 {
                    w353 = string[] [] ("pfade")
                    n201 = global write "musicplayer_glo.vi" "pfade"(w353) -> ()
                    n202 = property on="playlist" class="Listenfeld (strikt)"("Item Names"=w353, "Item Symbols"=i32[] [] ("Objektsymbole")) -> ()  [unwired: 2 in, 2 out]
                  }
                  frame #1 {
                    n203 = property on="playlist" class="Listenfeld (strikt)"("Top Row"=0 ("Erste Zeile")) -> ()  [unwired: 2 in, 2 out]
                  }
                }
              }
              frame "ADD_TITEL" {
                n204 = global read "musicplayer_glo.vi" "pfade"() -> (w362:string[])
                n205 = Index Array(array=w362, index=w360) -> (element=w364:string)
                n206 = property on="playlist" class="Listenfeld (strikt)"() -> ("Item Names"=w365:string[], "Item Symbols"=w356:i32[])  [unwired: 2 in, 2 out]
                n207 = global read "musicplayer_glo.vi" "Filetypes"() -> (w359:string)
                n208 = Not Equal?(x=w364, y="") -> (x != y?=w361:bool)
                n209 = call "add-titel.vi"("deutsch?"=w368, "abposeinfügen"=w361, "pfade"=w362, "use input-array?"=FALSE, "playlist"=w365, "symbole"=w356, "pos"=w360, "dateitypen"=w359) -> ("pfade out"=w367:string[], "playlist out"=w366:string[], "symbole out"=w355:dbl[])  [unwired: 5 in]
                n210 = global write "musicplayer_glo.vi" "pfade"(w367) -> ()
                n211 = property on="playlist" class="Listenfeld (strikt)"("Item Names"=w366, "Item Symbols"=w355) -> ()  [unwired: 2 in, 2 out]
              }
              frame "Tick all" {
                n212 = global read "musicplayer_glo.vi" "pfade"() -> (w370:string[])
                n213 = call "tickall.vi"("pfade"=w370) -> ("symbole out"=w369:dbl[])  [unwired: 10 in]
                n214 = property on="playlist" class="Listenfeld (strikt)"("Item Symbols"=w369) -> ()  [unwired: 2 in, 2 out]
              }
              frame "REMOVE_TITEL" {
                n215 = global read "musicplayer_glo.vi" "pfade"() -> (w374:string[])
                n216 = Index Array(array=w374, index=w372) -> (element=w376:string)
                n217 = Not Equal?(x=w376, y="") -> (x != y?=w373:bool)
                n218 = case shown="True" w373 {
                  tunnel: w374 -> [_ w383]
                  tunnel: w372 -> [_ w381]
                  frame False {
                  }
                  frame True {
                    n219 = property on="playlist" class="Listenfeld (strikt)"() -> ("Item Names"=w378:string[], "Item Symbols"=w377:i32[])  [unwired: 2 in, 2 out]
                    n220 = call "deletetitel.vi"("pos"=w381, "symbole"=w377, "playlist"=w378, "pfade"=w383) -> ("symbole out"=w380:dbl[], "playlist out"=w379:string[], "pfade out"=w382:string[])  [unwired: 5 in]
                    n221 = global write "musicplayer_glo.vi" "pfade"(w382) -> ()
                    n222 = property on="playlist" class="Listenfeld (strikt)"("Item Names"=w379, "Item Symbols"=w380) -> ()  [unwired: 2 in, 2 out]
                  }
                }
              }
              frame "REMOVE_NOT_AKTIVATED" {
                n223 = stacked-sequence {
                  frame #0 {
                    n224 = property on="playlist" class="Listenfeld (strikt)"() -> ("Item Names"=w387:string[], "Item Symbols"=w386:i32[])  [unwired: 2 in, 2 out]
                    n225 = global read "musicplayer_glo.vi" "pfade"() -> (w385:string[])
                    n226 = call "removenotticket.vi"("symbole"=w386, "playlist"=w387, "pfade"=w385) -> ("symbole out"=w390:dbl[], "playlist out"=w389:string[], "pfade out"=w388:string[])  [unwired: 6 in]
                    n227 = global write "musicplayer_glo.vi" "pfade"(w388) -> ()
                    n228 = property on="playlist" class="Listenfeld (strikt)"("Item Names"=w389, "Item Symbols"=w390) -> ()  [unwired: 2 in, 2 out]
                  }
                  frame #1 {
                    n229 = property on="playlist" class="Listenfeld (strikt)"("Top Row"=0 ("Erste Zeile")) -> ()  [unwired: 2 in, 2 out]
                  }
                }
              }
              frame "FOLLOW_PLAY" {
                n230 = call "Meldung an Benutzer"() -> ()  [unwired: 10 in, 2 out]
              }
            }
            n231 = case shown="True" w305 {
              frame False {
              }
              frame True {
                n232 = global read "musicplayer_glo.vi" "random?"() -> (w316:bool)
                n233 = case shown="True" w316 {
                  frame False {
                  }
                  frame True {
                    n234 = call "write_random_data.vi"() -> ()  [unwired: 12 in]
                  }
                }
              }
            }
          }
          event "playlist": Value Change {
            n235 = event-data() -> ("NewVal"=w399:i32[])  [unwired: 1 in]
            n236 = Array Size(array=w399) -> (size(s)=w400:i32)
            n237 = for {
              N: w400 -> [_]
              tunnel: w399 -> [w401]
              w407 = 37
              n238 = property on="playlist" class="Listenfeld (strikt)"() -> ("Item Symbols"=w408:i32[])  [unwired: 2 in, 2 out]
              n239 = Index Array(array=w401) -> (element=w403:i32)  [unwired: 1 in]
              n240 = Index Array(array=w408, index=w403) -> (element=w405:i32)
              n241 = Equal?(x=w405, y=w407) -> (x = y?=w404:bool)
              n242 = Select(t=38, s=w404, f=w407) -> (s? t:f=w409:i32)
              n243 = Replace Array Subset(array=w408, new element=w409, index=w403) -> (w402:i32[])
              n244 = property on="playlist" class="Listenfeld (strikt)"("Item Symbols"=w402) -> ()  [unwired: 2 in, 2 out]
            }
          }
          event Mouse Down {
            n245 = event-data() -> ()  [unwired: 1 in, 3 out]
            n246 = case shown="False" w412 {
              tunnel: w411 -> [_ w415]
              tunnel: [_ FALSE] -> w410
              frame False {
              }
              frame True {
                n247 = property on="playlist" class="Listenfeld (strikt)"("Active Row"=w415) -> ("CellBG"=w417:u32)  [unwired: 2 in, 2 out]
                n248 = Not Equal?(x=w417, y=u32 16382208 ("Farbfeld 2")) -> (x != y?=w416:bool)
                n249 = case shown="True" w416 {
                  tunnel: w415 -> [_ w419]
                  frame False {
                  }
                  frame True {
                    n250 = property on="playlist" class="Listenfeld (strikt)"("Active Row"=w419, "CellBG"=u32 65280 ("Farbfeld 2")) -> ()  [unwired: 2 in, 2 out]
                  }
                }
              }
            }
          }
          event Timeout {
            n251 = event-data() -> ()  [unwired: 1 in, 2 out]
            n252 = case shown="0, Standard" w421 {
              selector: w421 -> [_ w428]
              tunnel: [w424 w428] -> w420
              frame 0, Default {
                n253 = call "timeout.vi"() -> ("Time has Elapsed"=w425:bool)  [unwired: 12 in, 7 out]
                n254 = case shown="True" w425 {
                  tunnel: [_ 1] -> w424
                  frame False {
                  }
                  frame True {
                    n255 = local write "playlist"(i32[] [-1] ("playlist")) -> ()
                  }
                }
              }
              frame 1 {
              }
            }
          }
          event Panel Close? {
            n256 = event-data() -> ()  [unwired: 1 in, 2 out]
            n257 = global write "musicplayer_glo.vi" "playlist sichtbar?"(FALSE ("playlist sichtbar?")) -> ()
            n258 = event-data("Discard?"=TRUE ("Verwerfen?")) -> ()  [unwired: 1 in, 1 out]
          }
        }
        n259 = global read "musicplayer_glo.vi" "exit?"() -> (w261:bool)
      }
    }
    frame #4 {
      n260 = flat-sequence {
        tunnel: w433 -> [w435]
        frame #0 {
          n261 = local read "win msg queue"() -> (w434:T1)
          n262 = call "Destroy Windows Message Queue.vi"("win msg queue"=w434) -> ()  [unwired: 1 in, 1 out]
        }
        frame #1 {
          n263 = invoke class="VI" method="FP.Schließen"(reference=w435) -> ()  [unwired: 2 in, 3 out]
        }
      }
    }
  }
